vi "XY to Intensity Graph.vi"(8 "error in (no error)":errorcluster, 9 "Y Scale":dbl[](array[numeric]), 10 "Multiple XY-data in":cluster{"X-array":dbl[], "Y-array":dbl[]}[](array[cluster]) {"Y-array" format="%.2p"; "X-array" format="%.2p"}, 11 "graph_utilities in":refnum<class "graph_utilities.lvclass">) -> (0 "error out":errorcluster, 2 "Intensity Data":dbl[][](array[numeric]), 3 "graph_utilities out":refnum<class "graph_utilities.lvclass">)   [LabVIEW 2016, in "graph_utilities.lvclass"]
uses:
  graph_utilities.lvclass
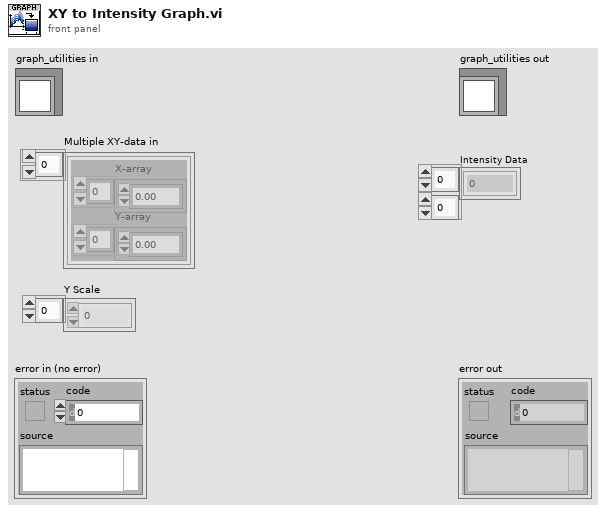
[diagram p1: front panel]
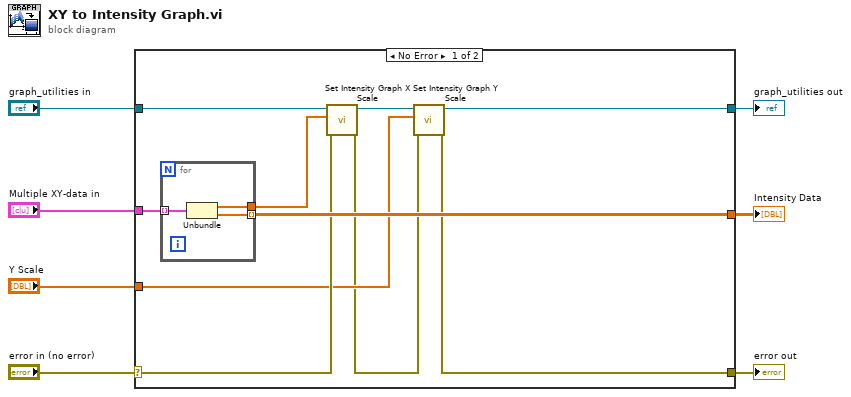
[diagram p0: block diagram]
diagram:
  n1 = case shown="No Error" "error in (no error)" {
    selector: "error in (no error)" -> [w14 w22]
    tunnel: [w8 w22] -> w6
    tunnel: [w10 w21] -> w4
    tunnel: "graph_utilities in" -> [w13 w21]
    tunnel: "Multiple XY-data in" -> [w17 _]
    tunnel: [w16 _] -> w2
    tunnel: "Y Scale" -> [w12 _]
    frame No Error {
      n2 = for {
        tunnel: w17 -> [w20] mode=indexing
        tunnel: [w19] -> w16 mode=indexing
        tunnel: [w18] -> w15
        n3 = Unbundle(w20) -> ("X-array"=w18:dbl[], "Y-array"=w19:dbl[])
      }
      n4 = call "Set Intensity Graph X Scale.vi"("error in (no error)"=w14, "X Scale"=w15, "graph_utilities in"=w13) -> ("error out"=w9:errorcluster, "graph_utilities out"=w11:refnum<class "graph_utilities.lvclass">)  [unwired: 7 in]
      n5 = call "Set Intensity Graph Y Scale.vi"("error in (no error)"=w9, "Y Scale"=w12, "graph_utilities in"=w11) -> ("error out"=w8:errorcluster, "graph_utilities out"=w10:refnum<class "graph_utilities.lvclass">)  [unwired: 7 in]
    }
    frame Error {
    }
  }
  "error out" <- w6
  "graph_utilities out" <- w4
  "Intensity Data" <- w2
